vi "OAT Polar PG Draw Polar Grids.vi"(5 "[user-specified font]":T3, 6 "channel settings":T1 {"probe angle [deg]" max=360 step=1; "shaft rotating direction" items=["CCW", "CW"]}, 7 "desired font(Application)":T5(ring)=enum."Application Font", 9 "polar attributes":T4 {"minimum" format="%.2f"; "maximum" format="%.2f"}, 10 "rect":T6={"left"=0, "top"=0, "right"=160, "bottom"=131}, 11 "picture":picture) -> (1 "grid measurements":T2 {"end angle" format="%.2f"; "start angle" format="%.2f"; "scale factors"."b" format="%.2f"; "scale factors"."a" format="%.2f"}, 3 "new picture":picture)   [LabVIEW 2017]
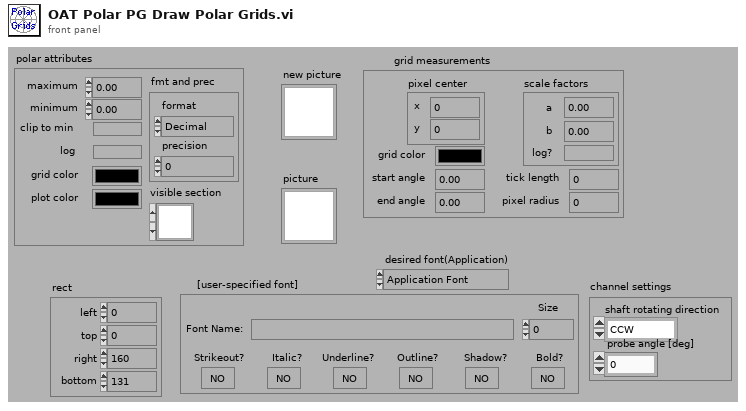
[diagram p1: front panel]
types:
  T1 = cluster{"shaft rotating direction":u16, "probe angle [deg]":u16}
  T2 = cluster{"pixel center":cluster{"x":i16, "y":i16}, "scale factors":cluster{"a":dbl, "b":dbl, "log?":bool}, "grid color":u32, "start angle":dbl, "end angle":dbl, "tick length":i16, "pixel radius":i32}
  T3 = cluster{"Font Name:":string, "Size":i16, "Strikeout?":bool, "Italic?":bool, "Underline?":bool, "Outline?":bool, "Shadow?":bool, "Bold?":bool}
  T4 = cluster{"maximum":dbl, "minimum":dbl, "clip to min":bool, "log":bool, "grid color":u32, "plot color":u32, "fmt and prec":cluster{"format":enum8{"Decimal", "Scientific", "Engineering", "Binary", "Octal", "Hex"}, "precision":u8}, "visible section":u16}
  T5 = enum16{"User-specified Font", "Application Font", "System Font", "Dialog Font"}
  T6 = cluster{"left":i16, "top":i16, "right":i16, "bottom":i16}
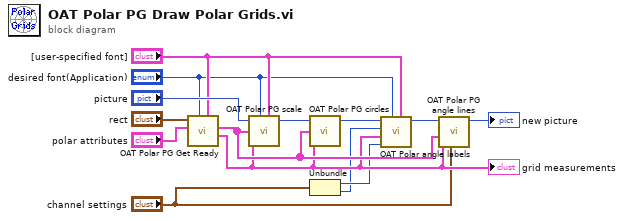
[diagram p0: block diagram]
diagram:
  n1 = call <vilib>:"OAT Polar PG Get Ready.vi"("polar attributes"="polar attributes", "rect"="rect", "desired font(Application)"="desired font(Application)", "[user-specified font]"="[user-specified font]") -> ("grid measurements"=w7:T2, "decade specs"=w12:cluster{"radius":i16, "label":string}[])  [unwired: 6 in]
  "grid measurements" <- w7
  n2 = call <vilib>:"OAT Polar PG scale.vi"("picture"="picture", "desired font(Application)"="desired font(Application)", "decade specs"=w12, "grid measurements"=w7, "[user-specified font]"="[user-specified font]") -> ("new picture"=w14:picture)  [unwired: 4 in]
  n3 = call <vilib>:"OAT Polar PG circles.vi"("picture"=w14, "decade specs"=w12, "grid measurements"=w7) -> ("new picture"=w8:picture)  [unwired: 6 in]
  n4 = Unbundle("channel settings") -> ("shaft rotating direction"=w4:u16, "probe angle [deg]"=w3:u16)
  n5 = call <vilib>:"OAT Polar angle labels.vi"("[user-specified font]"="[user-specified font]", "desired font(Application)"="desired font(Application)", "shaft rotating direction"=w4, "grid measurements"=w7, "probe position"=w3, "picture"=w8) -> ("new picture"=w2:picture)  [unwired: 5 in]
  n6 = call <vilib>:"OAT Polar PG angle lines.vi"("channel settings"="channel settings", "grid measurements"=w7, "decade specs"=w12, "picture"=w2) -> ("new picture"=→"new picture":picture)  [unwired: 7 in]
